vi "Stop Core.vi"(10 "final error code":i32, 11 "Nested in":refnum<class "Linear Encoder.lvclass">) -> (3 "Nested out":refnum<class "Linear Encoder.lvclass">)   [LabVIEW 2020, in "Linear Encoder.lvlib" / "Linear Encoder.lvclass"]
doc: "(<B>Filename</B>: Actor Framework.lvlib:Actor.lvclass:Stop Core.vi)\n\nDefines what the actor does before it stops. Use the <B>final error code</B> input to determine whether the actor shut down in response to an error.\n\nBy default, this method does nothing. A descendant class may override it to define behavior, such as shutting down any processes the actor initiated in its override of the Actor Core method."
uses:
  Linear Encoder.lvclass
  <vilib>/ActorFramework/Actor/Actor.lvclass
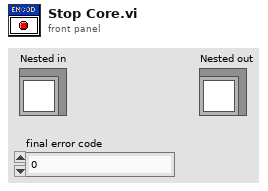
[diagram p1: front panel]
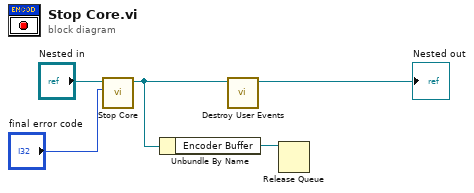
[diagram p0: block diagram]
diagram:
  n1 = call-parent "Stop Core.vi"("final error code"="final error code", "Actor in"="Nested in") -> ("Actor out"=w2:refnum<class "Linear Encoder.lvclass">)  [unwired: 9 in]
  n2 = Unbundle By Name(w2) -> ("Encoder Buffer"=w1:refnum<queue>)
  n3 = call "Destroy User Events.vi"("UI Template in"=w2) -> ("UI Template out"=→"Nested out":refnum<class "Linear Encoder.lvclass">)  [unwired: 10 in]
  n4 = Release Queue(queue=w1) -> ()  [unwired: 2 in, 3 out]
